vi "Msg To Nested.vi"(8 "Alias":string, 9 "Priority?":bool, 10 "Msg":refnum<class "Msg.lvclass">, 11 "jettl Queue Actor in":refnum<class "jettl Queue Actor.lvclass">) -> (0 "error out":errorcluster)   [LabVIEW 2021, in "jettl.lvlib" / "jettl Queue Actor.lvclass"]
uses:
  jettl Queue Actor.lvclass
  Actor/Msg/Msg.lvclass
  jettl Queue Actor.lvclass/jettl Queue Actor.ctl
  jettl.lvlib
panel:
  out "Nested Found?":bool
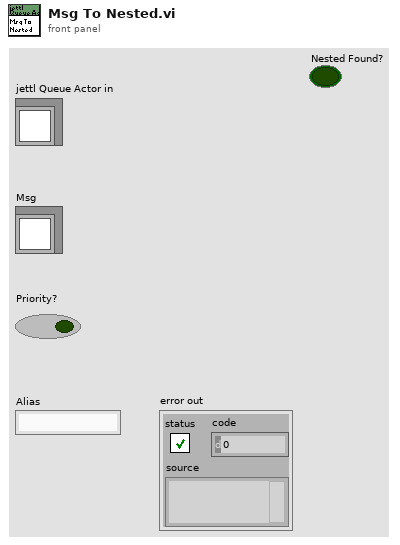
[diagram p1: front panel]
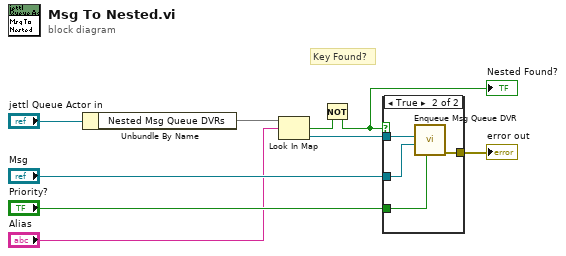
[diagram p0: block diagram]
diagram:
  # "Key Found?"
  n1 = Unbundle By Name("jettl Queue Actor in") -> ("Nested Msg Queue DVRs"=w5:map{string, refnum<data-value>})
  n2 = Look In Map(map=w5, key="Alias") -> (key not found?=w2:bool, value=w3:refnum<data-value>)  [unwired: 1 in]
  n3 = Not(x=w2) -> (.not. x?=w1:bool)
  "Nested Found?" <- w1
  n4 = case shown="True" w1 {
    tunnel: [_ w13] -> w9
    tunnel: "Msg" -> [_ w12]
    tunnel: "Priority?" -> [_ w11]
    tunnel: w3 -> [_ w10]
    frame False {
    }
    frame True {
      n5 = call "Enqueue Msg Queue DVR.vi"("Priority?"=w11, "Msg"=w12, "Msg Queue DVR"=w10) -> ("error out"=w13:errorcluster)  [unwired: 8 in]
    }
  }
  "error out" <- w9
